vi "test_spline.vi"() -> ()   [LabVIEW 2018]
uses:
  <vilib>/Analysis/NI_AALPro.lvlib
panel:
  out "Raw and Interpolated Data":T1(graph)
  in  "Original Data (X,Y)":dbl[][](array[numeric])=[[0.0, 1.0], [1.2, 2.700000047683716], [2.0, 7.400000095367432], [3.0, 150.0], [3.5, 140.0], [4.0, 80.0], [5.0, 220.0]] format="%0.2f"
  in  "Interpolation factor (n)":i32(slide)=4 scale=0.0..20.0
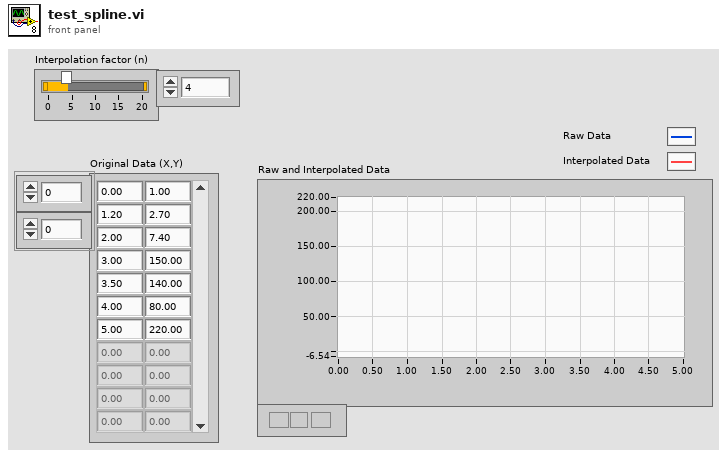
[diagram p1: front panel]
types:
  T1 = cluster{"Original Data (X,Y)":dbl[], "Original Data (X,Y)":dbl[]}[]
  T2 = enum16{"Linear", "Polynomial", "Spline", "Rational"}
  T3 = cluster{"Original Data (X,Y)":dbl[], "Original Data (X,Y)":dbl[]}
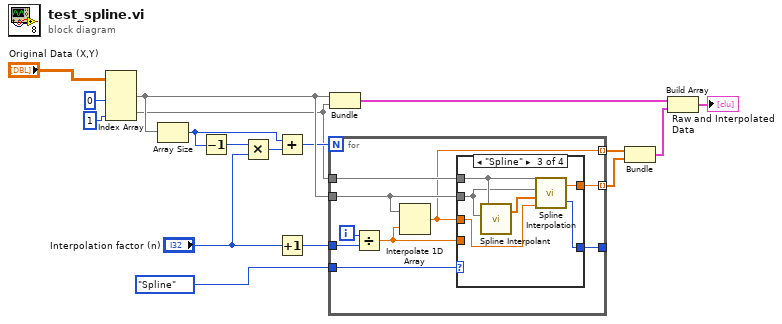
[diagram p0: block diagram]
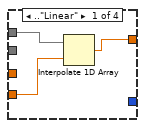
[diagram p2: hidden frame]
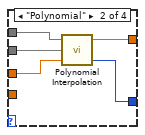
[diagram p3: hidden frame]
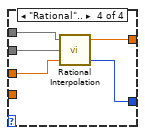
[diagram p4: hidden frame]
diagram:
  n1 = Index Array(array="Original Data (X,Y)", index (col) #1=0, index (col) #2=1 ("index (col)")) -> (element #1=w11:dbl[], element #2=w3:dbl[])  [unwired: 2 in]
  n2 = Array Size(array=w11) -> (size(s)=w7:i32)
  n3 = Decrement(x=w7) -> (x-1=w10:i32)
  n4 = Multiply(x=w10, y="Interpolation factor (n)") -> (x*y=w8:i32)
  n5 = Add(x=w7, y=w8) -> (x+y=w6:i32)
  n6 = Increment(x="Interpolation factor (n)") -> (x+1=w9:i32)
  n7 = for {
    N: w6 -> [_]
    tunnel: w3 -> [w26]
    tunnel: w11 -> [w20]
    tunnel: [w25] -> _
    tunnel: T2."Spline" ("Type of Interpolation") -> [w21]
    tunnel: w9 -> [w23]
    tunnel: [w22] -> w1 mode=indexing
    tunnel: [w19] -> w2 mode=indexing
    i -> [w24]
    n8 = Divide(x=w24, y=w23) -> (x/y=w18:dbl)
    n9 = Interpolate 1D Array(1:w18, 2:w20) -> (0:w19:dbl)
    n10 = case shown="\"Spline\"" w21 {
      tunnel: w19 -> [_ w34 w37 w41]
      tunnel: [w28 w33 w35 w43] -> w22
      tunnel: [_ w32 w36 w42] -> w25
      tunnel: w20 -> [_ w31 w38 w44]
      tunnel: w26 -> [w29 w30 w40 w45]
      tunnel: w18 -> [w27 _ _ _]
      frame .."Linear" {
        n11 = Interpolate 1D Array(1:w27, 2:w29) -> (0:w28:dbl)
      }
      frame "Polynomial" {
        n12 = call <vilib>:"Polynomial Interpolation.vi"("x value"=w34, "X"=w31, "Y"=w30) -> ("error"=w32:i32, "interpolation value"=w33:dbl)  [unwired: 1 out]
      }
      frame "Spline" {
        n13 = call <vilib>:"Spline Interpolant.vi"("X"=w38, "Y"=w40) -> ("Interpolant"=w39:dbl[])  [unwired: 2 in, 1 out]
        n14 = call <vilib>:"Spline Interpolation.vi"("x value"=w37, "Interpolant"=w39, "X"=w38, "Y"=w40) -> ("error"=w36:i32, "interpolation value"=w35:dbl)
      }
      frame "Rational".. {
        n15 = call <vilib>:"Rational Interpolation.vi"("x value"=w41, "X"=w44, "Y"=w45) -> ("error"=w42:i32, "interpolation value"=w43:dbl)  [unwired: 1 out]
      }
    }
  }
  n16 = Bundle("Original Data (X,Y)"=w11, "Original Data (X,Y)"=w3) -> (w12:T3)  [unwired: 1 in]
  n17 = Bundle(w2, w1) -> (w14:cluster{dbl[], dbl[]})  [unwired: 1 in]
  n18 = Build Array(w12, w14) -> (→"Raw and Interpolated Data":T1)
